vi "DO NOT RESCRIPT THIS MESSAGE.vi"(8 "error in (no error)":errorcluster, 11 "Event Handler Msg in":refnum<class "Event Handler Msg.lvclass">) -> (0 "error out":errorcluster, 3 "Event Handler Msg out":refnum<class "Event Handler Msg.lvclass">)   [LabVIEW 2026, in "TALOS.lvlib" / "Father of all uServices.lvlib" / "Event Handler Msg.lvclass"]
uses:
  Event Handler Msg.lvclass
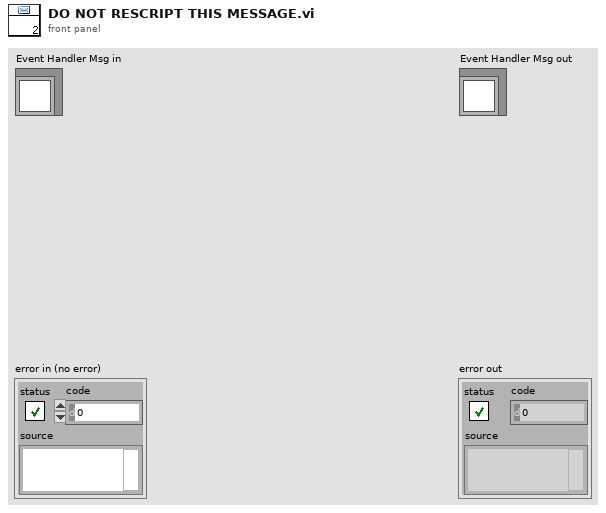
[diagram p1: front panel]
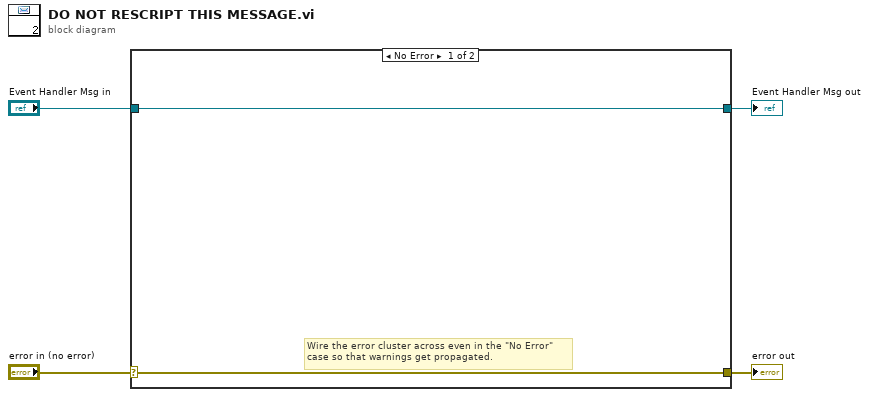
[diagram p0: block diagram]
diagram:
  n1 = case shown="No Error" "error in (no error)" {
    selector: "error in (no error)" -> [w5 w8]
    tunnel: [w5 w8] -> w3
    tunnel: [w6 w7] -> w1
    tunnel: "Event Handler Msg in" -> [w6 w7]
    frame No Error {
      # "Wire the error cluster across even in the \"No Error\"\ncase so that warnings get propagated."
    }
    frame Error {
    }
  }
  "error out" <- w3
  "Event Handler Msg out" <- w1
